vi "Match Wildcard Pattern String List.vi"(3 "case matching (sensitive)":T1=enum."system", 4 "pattern":string, 5 "string list":string[](array[string])=["lybraryn.llb/*", "memmon.llb/*"]) -> (0 "found pattern":bool, 1 "string":string, 2 "index":i32)   [LabVIEW 2015, in "TLB` Template.lvlib" / "Tools_String.lvlib"]
doc: "TLB Prime - Application Template 1.3.0.24\nNorm Kirchner, NI Systems Engineering - NI\nCopyright (c) 2014, NI"
uses:
  Tools_String.lvlib
  <vilib>/FTP/util/Case Matching.ctl
  Get Case Insensitive Search Pattern.vi
  Get Wildcard Search Pattern.vi
  <vilib>/FTP/NI_FTP.lvlib
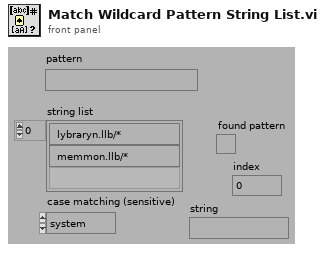
[diagram p1: front panel]
types:
  T1 = typedef "NI_FTP.lvlib/Case Matching.ctl" = enum16{"a != A", "a == A", "system"}
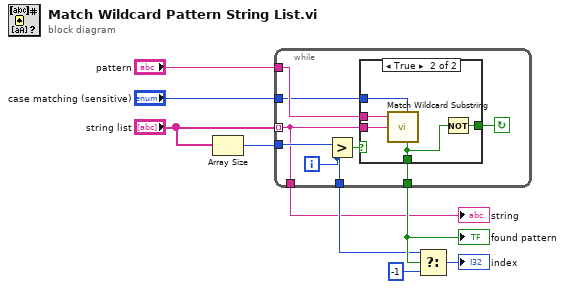
[diagram p0: block diagram]
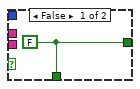
[diagram p2: hidden frame]
diagram:
  n1 = Array Size(array="string list") -> (size(s)=w7:i32)
  n2 = while {
    tunnel: [w11] -> w2
    tunnel: [w13] -> w4
    tunnel: [w15] -> w6
    tunnel: "pattern" -> [w12]
    tunnel: w7 -> [w17]
    tunnel: "string list" -> [w11] mode=indexing
    tunnel: "case matching (sensitive)" -> [w10]
    i -> [w13]
    stop <- w14 continue-if-true
    n3 = Greater?(x=w17, y=w13) -> (0:w16:bool)
    n4 = case shown="True" w16 {
      tunnel: w11 -> [_ w21]
      tunnel: [w18 w23] -> w15
      tunnel: [w18 w22] -> w14
      tunnel: w12 -> [_ w20]
      tunnel: w10 -> [_ w19]
      frame False {
        w18 = FALSE
      }
      frame True {
        n5 = call "Match Wildcard Substring.vi"("case matching (sensitive)"=w19, "string"=w21, "pattern with wildcards"=w20) -> ("found substring"=w23:bool)  [unwired: 1 in, 4 out]
        n6 = Not(x=w23) -> (.not. x?=w22:bool)
      }
    }
  }
  "found pattern" <- w6
  "string" <- w2
  n7 = Select(t=w4, s=w6, f=-1) -> (s? t:f=→"index":i32)
